vi "Initialize Device.vi"(0 "Device in":refnum<class "Device.lvclass">, 5 "error in":errorcluster) -> (14 "Device out":refnum<class "Device.lvclass">, 19 "error out":errorcluster)   [LabVIEW 2014, in "DAQ Device.lvlib" / "Device.lvclass"]
uses:
  Device.lvclass
  Device.lvclass/Device.ctl
  Controller/xGlobal Data.vi
  Devices/Configurable Device/Configurable Device.lvclass
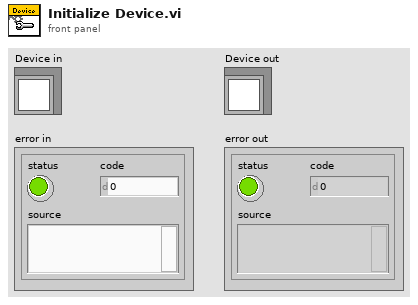
[diagram p1: front panel]
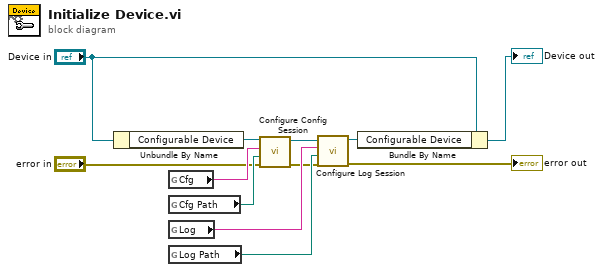
[diagram p0: block diagram]
diagram:
  n1 = Unbundle By Name("Device in") -> ("Configurable Device"=w7:refnum<class "Configurable Device.lvclass">)
  n2 = global read "xGlobal Data.vi" "Cfg"() -> (w11:string)
  n3 = global read "xGlobal Data.vi" "Cfg Path"() -> (w12:path)
  n4 = global read "xGlobal Data.vi" "Log"() -> (w10:string)
  n5 = global read "xGlobal Data.vi" "Log Path"() -> (w9:path)
  n6 = call "Configure Config Session.vi"("error in"="error in", "Path"=w12, "Ref Name"=w11, "Configurable Device in"=w7) -> ("error out"=w6:errorcluster, "Configurable Device out"=w5:refnum<class "Configurable Device.lvclass">)  [unwired: 6 in]
  n7 = call "Configure Log Session.vi"("error in"=w6, "Path"=w9, "Ref Name"=w10, "Configurable Device in"=w5) -> ("error out"=→"error out":errorcluster, "Configurable Device out"=w3:refnum<class "Configurable Device.lvclass">)  [unwired: 6 in]
  n8 = Bundle By Name(cluster="Device in", "Configurable Device"=w3) -> (→"Device out":refnum<class "Device.lvclass">)
